vi "BuildClass.vi"(7 "Parent":enum16{"None", "Interface", "Class"}(ring), 8 "error in (no error)":errorcluster, 11 "CreateClass in":refnum<class "CreateClass.lvclass">) -> (0 "error out":errorcluster, 3 "CreateClass Out":refnum<class "CreateClass.lvclass">)   [LabVIEW 2020, in "Mermaid.lvlib" / "CreateClass.lvclass"]
uses:
  CreateClass.lvclass
  CreateClass.lvclass/CreateClass.ctl
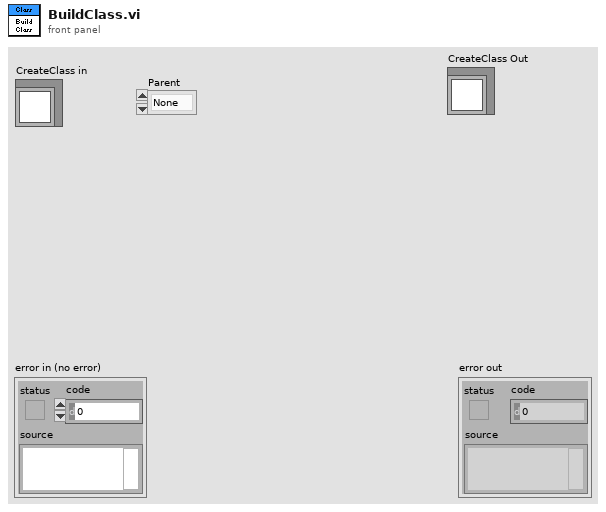
[diagram p1: front panel]
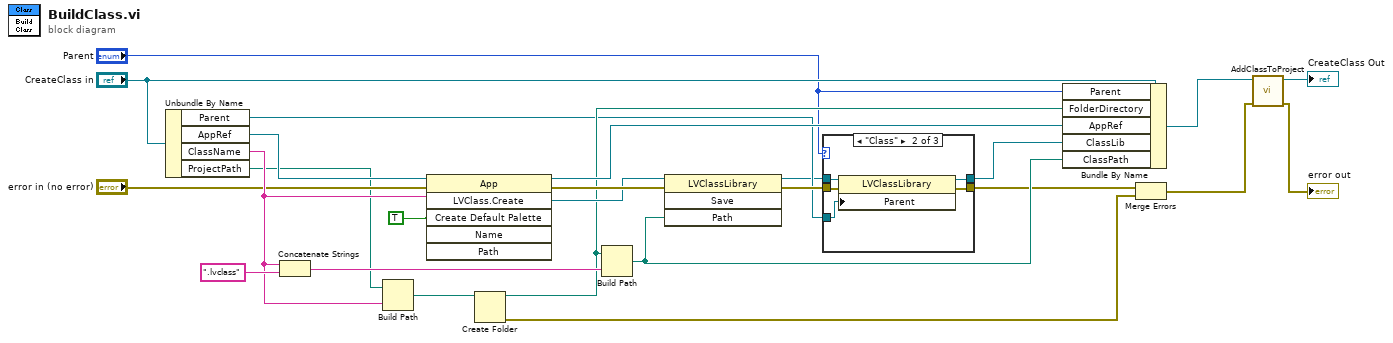
[diagram p0: block diagram]
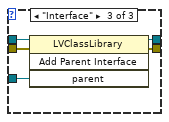
[diagram p3: hidden frame]
diagram:
  n1 = Unbundle By Name("CreateClass in") -> ("Parent"=w5:refnum<vi>, "AppRef"=w19:refnum<vi>, "ClassName"=w18:string, "ProjectPath"=w1:path)
  n2 = Concatenate Strings(w18, ".lvclass" ("string")) -> (w23:string)
  n3 = Build Path(base path=w1, name or relative path=w18) -> (appended path=w21:path)
  n4 = invoke class="App" method="LVClass.Create"(reference=w19, error in="error in (no error)", "Create Default Palette"=TRUE ("Create:Default Palette"), "Name"=w18) -> (reference out=w17:refnum<vi>, error out=w22:errorcluster, "LVClass.Create"=w20:refnum<vi>)  [unwired: 2 in, 3 out]
  n5 = Create Folder(path (use dialog)=w21) -> (created path=w14:path, error out=w15:errorcluster)  [unwired: 2 in, 1 out]
  n6 = Build Path(base path=w14, name or relative path=w23) -> (appended path=w13:path)
  n7 = invoke class="LVClassLibrary" method="Save"(reference=w20, error in=w22, "Path"=w13) -> (reference out=w4:refnum<vi>, error out=w7:errorcluster)  [unwired: 1 in, 2 out]
  n8 = case shown="\"Class\"" "Parent" {
    tunnel: w4 -> [w26 w32 w37]
    tunnel: w7 -> [w27 w31 w36]
    tunnel: [w26 w30 w35] -> w3
    tunnel: [w27 w29 w34] -> w6
    tunnel: w5 -> [_ w28 w33]
    frame "None", Default {
    }
    frame "Class" {
      n9 = property class="LVClassLibrary"(reference=w32, error in=w31, "Parent"=w28) -> (reference out=w30:refnum<vi>, error out=w29:errorcluster)
    }
    frame "Interface" {
      n10 = invoke class="LVClassLibrary" method="Add Parent Interface"(reference=w37, error in=w36, "parent"=w33) -> (reference out=w35:refnum<vi>, error out=w34:errorcluster)  [unwired: 1 in, 2 out]
    }
  }
  n11 = Bundle By Name(cluster="CreateClass in", "Parent"="Parent", "FolderDirectory"=w14, "AppRef"=w17, "ClassLib"=w3, "ClassPath"=w13) -> (w11:refnum<class "CreateClass.lvclass">)
  n12 = Merge Errors(w6, w15) -> (w10:errorcluster)
  n13 = call "AddClassToProject.vi"("error in (no error)"=w10, "CreateClass In"=w11) -> ("error out"=→"error out":errorcluster, "CreateClass Out"=→"CreateClass Out":refnum<class "CreateClass.lvclass">)  [unwired: 8 in]
